vi "SetOperationRunStartTime.vi"(8 "error in":errorcluster, 10 "OperationRunStartTime":timestamp, 11 "OperationRun in":refnum<class "OperationRun.lvclass">) -> (0 "error out":errorcluster, 3 "OperationRun out":refnum<class "OperationRun.lvclass">)   [LabVIEW 2021, in "ProligentXMLGenerator.lvlib" / "OperationRun.lvclass"]
doc: "Defines the start date of the operation run.\n\nThis value is limited to 2000 charactesrs and must no be empty."
uses:
  OperationRun.lvclass
  OperationRun.lvclass/OperationRun.ctl
  Base/DateTime/DateTime.lvclass
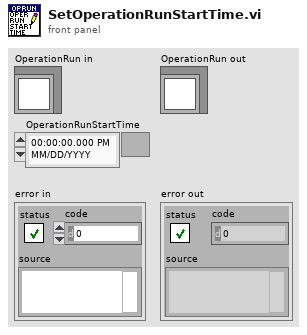
[diagram p1: front panel]
types:
  T1 = typedef "ProligentXMLGenerator.lvlib/OperationRun.lvclass/Data.ctl" = cluster{"Name":string, "Characteristics":refnum<class "Characteristic.lvclass">[], "Documents":refnum<class "Document.lvclass">[], "SequenceRuns":refnum<class "SequenceRun.lvclass">[], "FailureReferences":refnum<class "FailureReference.lvclass">[], "SequenceRunReferences":refnum<class "SequenceRunReference.lvclass">[], "CustomData":refnum<class "CustomData.lvclass">, "OperationRunId":refnum<class "Guid.lvclass">, "ProcessFullName":refnum<class "ProcessFullName.lvclass">, "ProcessVersion":refnum<class "NonEmptyString_64.lvclass">, "OperationName":refnum<class "NonEmptyString_65.lvclass">, "StationFullName":refnum<class "FullName.lvclass">, "User":refnum<class "NonEmptyString_255.lvclass">, "CallingOperationRunId":refnum<class "Guid.lvclass">, "OperationStatus":refnum<class "ExecutionStatus.lvclass">, "OperationRunStartTime":refnum<class "DateTime.lvclass">, "OperationRunEndTime":refnum<class "DateTime.lvclass">, "TimeZoneInfoId":string}
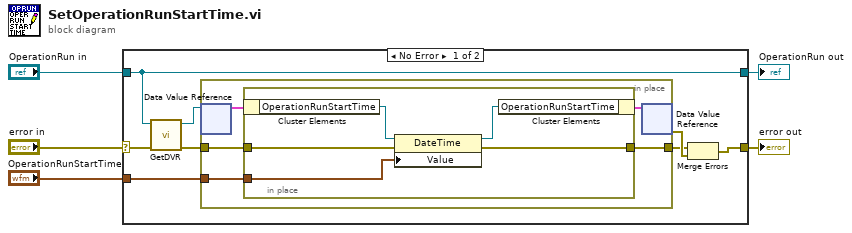
[diagram p0: block diagram]
diagram:
  n1 = case shown="No Error" "error in" {
    selector: "error in" -> [w11 w24]
    tunnel: "OperationRun in" -> [w6 w25]
    tunnel: [w8 w24] -> w3
    tunnel: "OperationRunStartTime" -> [w7 _]
    tunnel: [w6 w25] -> w1
    frame No Error {
      n2 = call "GetDVR.vi"("error in"=w11, "OperationRun"=w6) -> ("error out"=w10:errorcluster, "DVRReference"=w12:refnum<data-value>)  [unwired: 8 in]
      n3 = in-place "In Place Element Structure" {
        in-place-border: w10 -> [w18]
        in-place-border: [w17] -> w9
        in-place-border: w7 -> [w16]
        n4 = in-place-dvr #1(w12) -> (w15:T1)  [unwired: 1 out]
        n5 = in-place "In Place Element Structure" {
          in-place-border: w18 -> [w23]
          in-place-border: [w22] -> w17
          in-place-border: w16 -> [w21]
          n6 = in-place-cluster #2(w15) -> ("OperationRunStartTime"=w20:refnum<class "DateTime.lvclass">)
          n7 = property on="Property Node" class="DateTime"(reference=w20, error in=w23, "Value"=w21) -> (reference out=w19:refnum<class "DateTime.lvclass">, error out=w22:errorcluster)
          n8 = in-place-cluster #2("OperationRunStartTime"=w19) -> (w14:T1)
        }
        n9 = in-place-dvr #1(w14) -> (w13:errorcluster)  [unwired: 1 out]
      }
      n10 = Merge Errors(w9, w13) -> (w8:errorcluster)
    }
    frame Error {
    }
  }
  "error out" <- w3
  "OperationRun out" <- w1
